vi "Configure Measurement Filter.vi"(5 "Window":dbl=0.1 max=10.0, 6 "Number of Filter Readings (10)":u32=10 min=1 max=100, 7 "Filter Type":u16(ring) items=["Repeating", "Moving"], 8 "error in (no error)":errorcluster, 9 "Enable Filter  (T: Enable)":bool=TRUE, 10 "Function":u16(ring) items=["Voltage: DC", "Voltage: AC", "Current: DC", "Current: AC", "2W Resistance", "4W Resistance", "Diode", "Capacitance", "Temperature", "Continuity", "Frequency", "Period", "Ratio", "Digitize Voltage", "Digitize Current"], 11 "VISA resource name":refnum<visa-resource-name>) -> (0 "error out":errorcluster, 3 "VISA resource name out":refnum<visa-resource-name>)   [LabVIEW 2021, in "Keithley DMM7510.lvlib"]
doc: "Configures the measurement filter, including the number of readings averaged the type of filter applied."
uses:
  Keithley DMM7510.lvlib
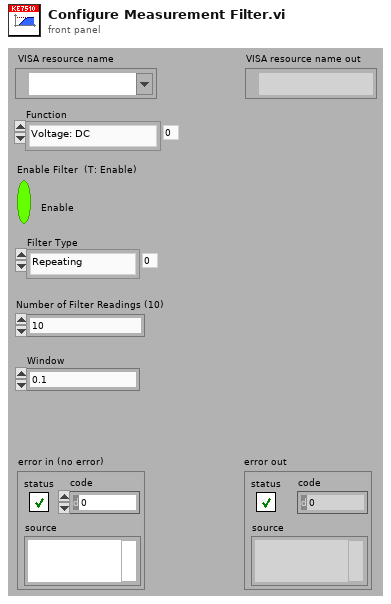
[diagram p1: front panel]
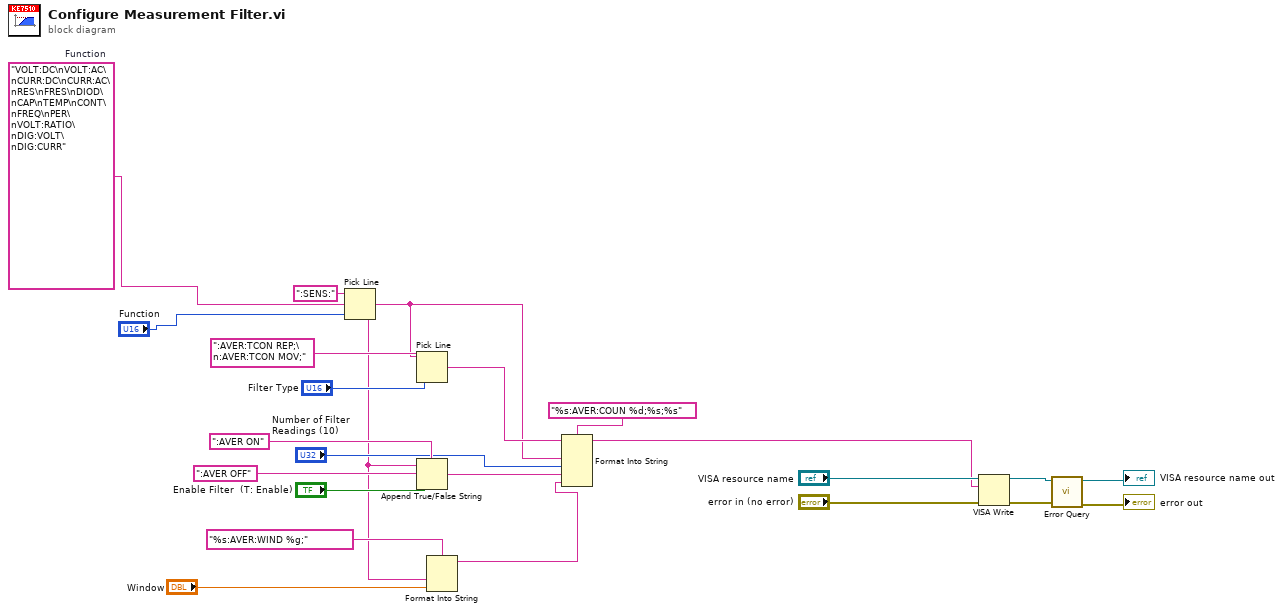
[diagram p0: block diagram]
diagram:
  w2 = "VOLT:DC\nVOLT:AC\nCURR:DC\nCURR:AC\nRES\nFRES\nDIOD\nCAP\nTEMP\nCONT\nFREQ\nPER\nVOLT:RATIO\nDIG:VOLT\nDIG:CURR"  # Function
  n1 = Pick Line(string ("")=":SENS:", multi-line string=w2, line index="Function") -> (output string=w10:string)
  n2 = Pick Line(string ("")=w10, multi-line string=":AVER:TCON REP;\n:AVER:TCON MOV;", line index="Filter Type") -> (output string=w12:string)
  n3 = Append True/False String(1:"Enable Filter  (T: Enable)", 2:":AVER OFF", 3:":AVER ON", 4:w10) -> (0:w14:string)
  n4 = Format Into String(format string="%s:AVER:WIND %g;", w10, "Window") -> (resulting string=w8:string)  [unwired: 2 in, 1 out]
  n5 = Format Into String(format string="%s:AVER:COUN %d;%s;%s", initial string=w12, w10, "Number of Filter Readings (10)", w14, w8) -> (resulting string=w18:string)  [unwired: 1 in, 1 out]
  n6 = VISA Write(VISA resource name="VISA resource name", write buffer=w18, error in (no error)="error in (no error)") -> (VISA resource name out=w7:refnum<visa-resource-name>, error out=w6:errorcluster)  [unwired: 1 out]
  n7 = call "Error Query.vi"("error in (no error)"=w6, "VISA resource name"=w7) -> ("error out"=→"error out":errorcluster, "VISA resource name out"=→"VISA resource name out":refnum<visa-resource-name>)  [unwired: 8 out]
